vi "Close.vi"(8 "error in (no error)":errorcluster, 11 "ControlClassWizard in":refnum<class "QControl Creation Wizard.lvclass">) -> (0 "error out":errorcluster)   [LabVIEW 2020, in "QControl Creation Wizard.lvclass"]
doc: "<b> </b> <b> </b>\n©2016 Q Software Innovations, LLC (QSI)\nwritten by Quentin Alldredge\nproduced in LabVIEW 2015\n\nsupport@qsoftwareinnovations.com\nwww.qsoftwareinnovations.com\n\nAll rights reserved.\n\nRedistribution and use in source and binary forms, with or without modification, are permitted provided that the following conditions are met:\n\n * Redistributions of source code must retain the above copyright notice, this list of conditions and the following disclaimer.\n * Redistributions in binary form must reproduce the above copyright notice, this list of conditions and the following disclaimer in the documentation and/or other materials provided with the distribution.\n * Neither the name of Q Software Innovations, LLC. nor the names of its contributors may be used to endorse or promote products derived from this software without specific prior written permission.\n\nTHIS SOFTWARE IS PROVIDED BY THE COPYRIGHT HOLDERS AND CONTRIBUTORS \"AS IS\" AND ANY EXPRESS OR IMPLIED WARRANTIES, INCLUDING, BUT NOT LIMITED TO, THE IMPLIED WARRANTIES OF MERCHANTABILITY AND FITNESS FOR A PARTICULAR PURPOSE ARE DISCLAIMED. IN NO EVENT SHALL THE COPYRIGHT OWNER OR CONTRIBUTORS BE LIABLE FOR ANY DIRECT, INDIRECT, INCIDENTAL, SPECIAL, EXEMPLARY, OR CONSEQUENTIAL DAMAGES (INCLUDING, BUT NOT LIMITED TO, PROCUREMENT OF SUBSTITUTE GOODS OR SERVICES; LOSS OF USE, DATA, OR PROFITS; OR BUSINESS INTERRUPTION) HOWEVER CAUSED AND ON ANY THEORY OF LIABILITY, WHETHER IN CONTRACT, STRICT LIABILITY, OR TORT (INCLUDING NEGLIGENCE OR OTHERWISE) ARISING IN ANY WAY OUT OF THE USE OF THIS SOFTWARE, EVEN IF ADVISED OF THE POSSIBILITY OF SUCH DAMAGE."
uses:
  QControl Creation Wizard.lvclass
  C:/ODP/QControlToolkit/QControl Wizard/QControl Creation Wizard/Dialog/Dialog.lvclass
  QControl Creation Wizard.lvclass/QControl Creation Wizard.ctl
  Dialog/Dialog.lvclass
  QControl Classes/TreeSelectionSingle/TreeSelectionSingle.lvclass
  QControl Classes/Steps/Steps.lvclass
  QControl Classes/StatusHistory/StatusHistory.lvclass
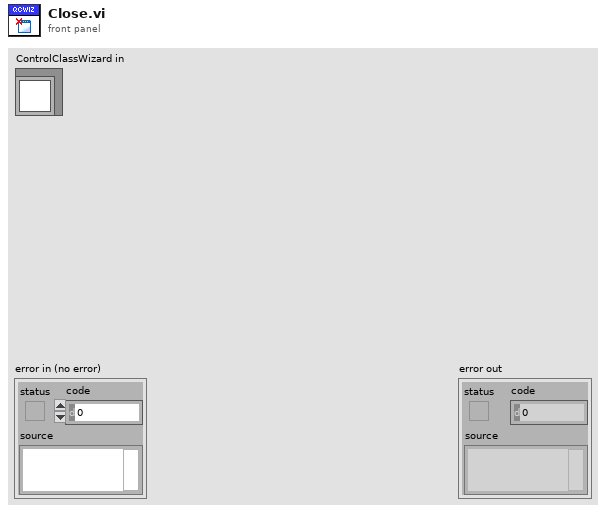
[diagram p1: front panel]
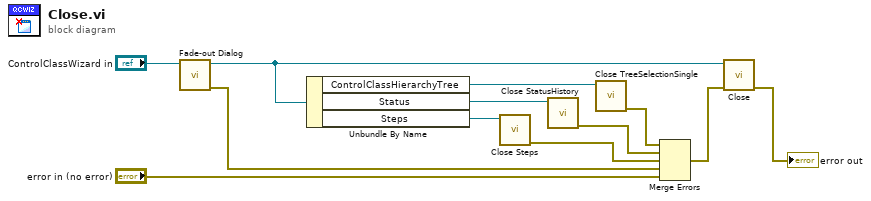
[diagram p0: block diagram]
diagram:
  n1 = call "Fade-out Dialog.vi"("Dialog in"="ControlClassWizard in") -> ("error out"=w9:errorcluster, "Dialog out"=w10:refnum<class "QControl Creation Wizard.lvclass">)  [unwired: 9 in]
  n2 = Unbundle By Name(w10) -> ("ControlClassHierarchyTree"=w8:refnum<class "TreeSelectionSingle.lvclass">, "Status"=w4:refnum<class "StatusHistory.lvclass">, "Steps"=w6:refnum<class "Steps.lvclass">)
  n3 = call "Close Steps.vi"("Steps in"=w6) -> ("error out"=w5:errorcluster)  [unwired: 9 in, 1 out]
  n4 = call "Close StatusHistory.vi"("StatusHistory in"=w4) -> ("error out"=w3:errorcluster)  [unwired: 10 in]
  n5 = call "Close TreeSelectionSingle.vi"("TreeSelectSingle in"=w8) -> ("error out"=w7:errorcluster)  [unwired: 10 in]
  n6 = Merge Errors(w7, w3, w5, w9, "error in (no error)") -> (w1:errorcluster)
  n7 = call-parent "Close.vi"("error in (no error)"=w1, "Dialog in"=w10) -> ("error out"=→"error out":errorcluster)  [unwired: 9 in]
